vi "Prepare Joystick Data for Displays.vi"(11 "Joystick Values":T2) -> (0 "Hat Switch Cluster":T1, 1 "Buttons":T3, 2 "Z Axis":dbl, 3 "Cartesian Data":cluster{"X axis":dbl, "X axis":dbl}[](array[cluster]), 6 "Axis 4":dbl)   [LabVIEW 2015]
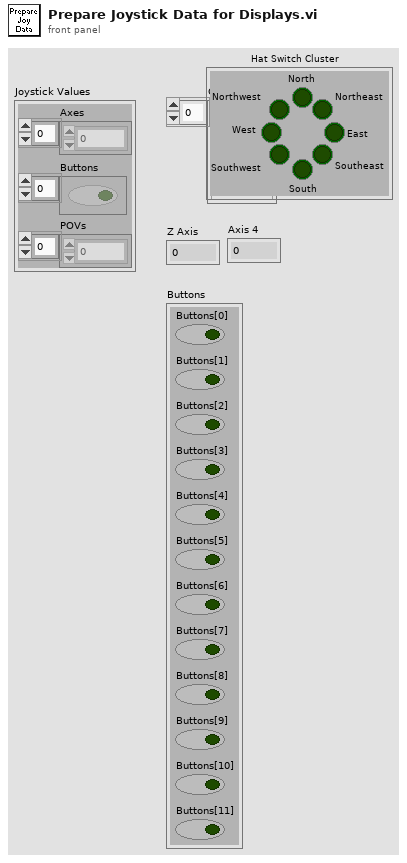
[diagram p1: front panel]
types:
  T1 = cluster{"North":bool, "Northeast":bool, "East":bool, "Southeast":bool, "South":bool, "Southwest":bool, "West":bool, "Northwest":bool}
  T2 = cluster{"Axes":dbl[], "Buttons":bool[], "POVs":i16[]}
  T3 = cluster{"Buttons[0]":bool, "Buttons[1]":bool, "Buttons[2]":bool, "Buttons[3]":bool, "Buttons[4]":bool, "Buttons[5]":bool, "Buttons[6]":bool, "Buttons[7]":bool, "Buttons[8]":bool, "Buttons[9]":bool, "Buttons[10]":bool, "Buttons[11]":bool}
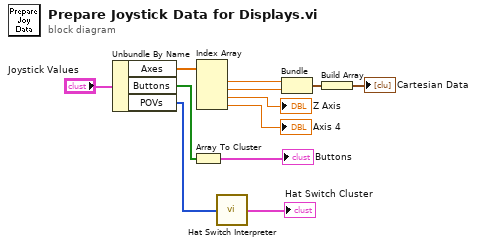
[diagram p0: block diagram]
diagram:
  n1 = Unbundle By Name("Joystick Values") -> ("Axes"=w5:dbl[], "Buttons"=w11:bool[], "POVs"=w3:i16[])
  n2 = Array To Cluster(array=w11) -> (cluster=→"Buttons":T3)
  n3 = Index Array(array=w5) -> (element #1=w8:dbl, element #2=w9:dbl, element #3=→"Z Axis":dbl, element #4=→"Axis 4":dbl)  [unwired: 4 in]
  n4 = call "Hat Switch Interpreter.vi"("POVs"=w3) -> ("Hat Switch Cluster"=→"Hat Switch Cluster":T1)  [unwired: 4 out]
  n5 = Bundle("X axis"=w8, "X axis"=w9) -> (w7:cluster{"X axis":dbl, "X axis":dbl})  [unwired: 1 in]
  n6 = Build Array(w7) -> (→"Cartesian Data":cluster{"X axis":dbl, "X axis":dbl}[])
